vi "Periodic Tasks.vi"(8 "error in":errorcluster) -> ()   [LabVIEW 2015]
doc: "This VI runs in parallel to other tasks. It can contain as many user-defined periodic loops as you need. These can carry out PID or other sorts of timed response."
uses:
  <vilib>/Rock Robotics/WPI/Solenoid/WPI_SolenoidValue.ctl
  Robot Global Data.vi
  <vilib>/Rock Robotics/Network Tables/NT Write Raw.vi
  <vilib>/Rock Robotics/Network Tables/NT Write Boolean.vi
  <vilib>/Rock Robotics/WPI/Solenoid/WPI_SolenoidSetEnum.vi
  <vilib>/Rock Robotics/Network Tables/NT Write Number.vi
  <vilib>/Rock Robotics/Network Tables/NT Write Numeric Array.vi
  <vilib>/Rock Robotics/Network Tables/NT Read Boolean.vi
  <vilib>/Rock Robotics/WPI/Utilities/WPI_GetSetVariantRefNum.vi
panel:
  in  "Trim Speed":dbl
  in  "Rate":dbl min=0.0 max=0.1 step=0.001
  out "Ramp Up":dbl(knob) scale=0.0..1.0
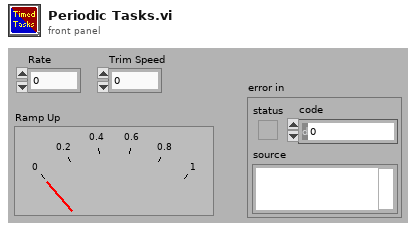
[diagram p1: front panel]
types:
  T1 = typedef "WPI_SolenoidValue.ctl" = enum16{"Off", "On", "Forward", "Reverse"}
  T2 = typedef "WPI_MotorControlDeviceRef.ctl" = cluster{"DeviceStatus":errorcluster, "Type":T3, "PWM":cluster{"PWM Channel":T4, "DeadBand":T5}, "CAN":cluster{"Device Number":u8, "Control Mode":T6, "Semaphore":T7, "Max Vout":dbl, "TalonSRX Control Mode":T8}, "Invert":bool}
  T3 = typedef "WPI_MotorControlType.ctl" = enum16{"PWM", "CAN", "CANTalonSRX"}
  T4 = typedef "FPGA_DIOPWMChannel.ctl" = enum8{"PWM 0", "PWM 1", "PWM 2", "PWM 3", "PWM 4", "PWM 5", "PWM 6", "PWM 7", "PWM 8", "PWM 9", "PWM MXP 0", "PWM MXP 1", "PWM MXP 2", "PWM MXP 3", "PWM MXP 4", "PWM MXP 5", "PWM MXP 6", "PWM MXP 7", "PWM MXP 8", "PWM MXP 9", "Invalid"}
  T5 = typedef "WPI_PWMDeadband.ctl" = cluster{"Name":string, "maxPositivePwm":i32, "minPositivePwm":i32, "centerPwm":i32, "maxNegativePwm":i32, "minNegativePwm":i32, "angularRange":u16}
  T6 = typedef "WPI_CANJaguar_ControlMode.ctl" = enum8{"Percent VBus", "Current", "Speed", "Position", "Voltage"}
  T7 = typedef "Semaphore RefNum" = refnum<k1>
  T8 = typedef "WPI_CANTalonSRX_APIControlMode.ctl" = enum8{"Percent VBus", "Speed", "Position", "Slave", "Unchanged / Invalid", "Voltage Compensation", "Current", "Motion Profile"}
  T9 = typedef "WPI_SolenoidDevRef.ctl" = cluster{"DevStatus":errorcluster, "Pneumatics Control Module":u8, "Forward Solenoid Channel":T10, "Reverse Solenoid Channel":T10}
  T10 = typedef "WPI_SolenoidChannel.ctl" = enum8{"Solenoid 0", "Solenoid 1", "Solenoid 2", "Solenoid 3", "Solenoid 4", "Solenoid 5", "Solenoid 6", "Solenoid 7", "Invalid"}
  T11 = typedef "WPI_DigitalInputDevRef.ctl" = cluster{"DevStatus":errorcluster, "DIO Channel":T12}
  T12 = typedef "FPGA_DIOChannel.ctl" = enum8{"DIO 0", "DIO 1", "DIO 2", "DIO 3", "DIO 4", "DIO 5", "DIO 6", "DIO 7", "DIO 8", "DIO 9", "DIO MXP 0", "DIO MXP 1", "DIO MXP 2", "DIO MXP 3", "DIO MXP 4", "DIO MXP 5", "DIO MXP 6", "DIO MXP 7", "DIO MXP 8", "DIO MXP 9", "DIO MXP 10", "DIO MXP 11", "DIO MXP 12", "DIO MXP 13", "DIO MXP 14", "DIO MXP 15", "Invalid"}
  T13 = typedef "WPI_RobotDriveDevRef.ctl" = cluster{"DevStatus":errorcluster, "Motors[]":T2[], "Square Inputs":bool, "Max Output":dbl}
  T14 = typedef "WPI_DriverStationRobotMode2.ctl" = enum16{"Autonomous Disabled", "Autonomous Enabled", "Teleop Disabled", "Teleop Enabled", "Disconnected", "Finish", "Test Disabled", "Test Enabled", "Emergency Stopped"}
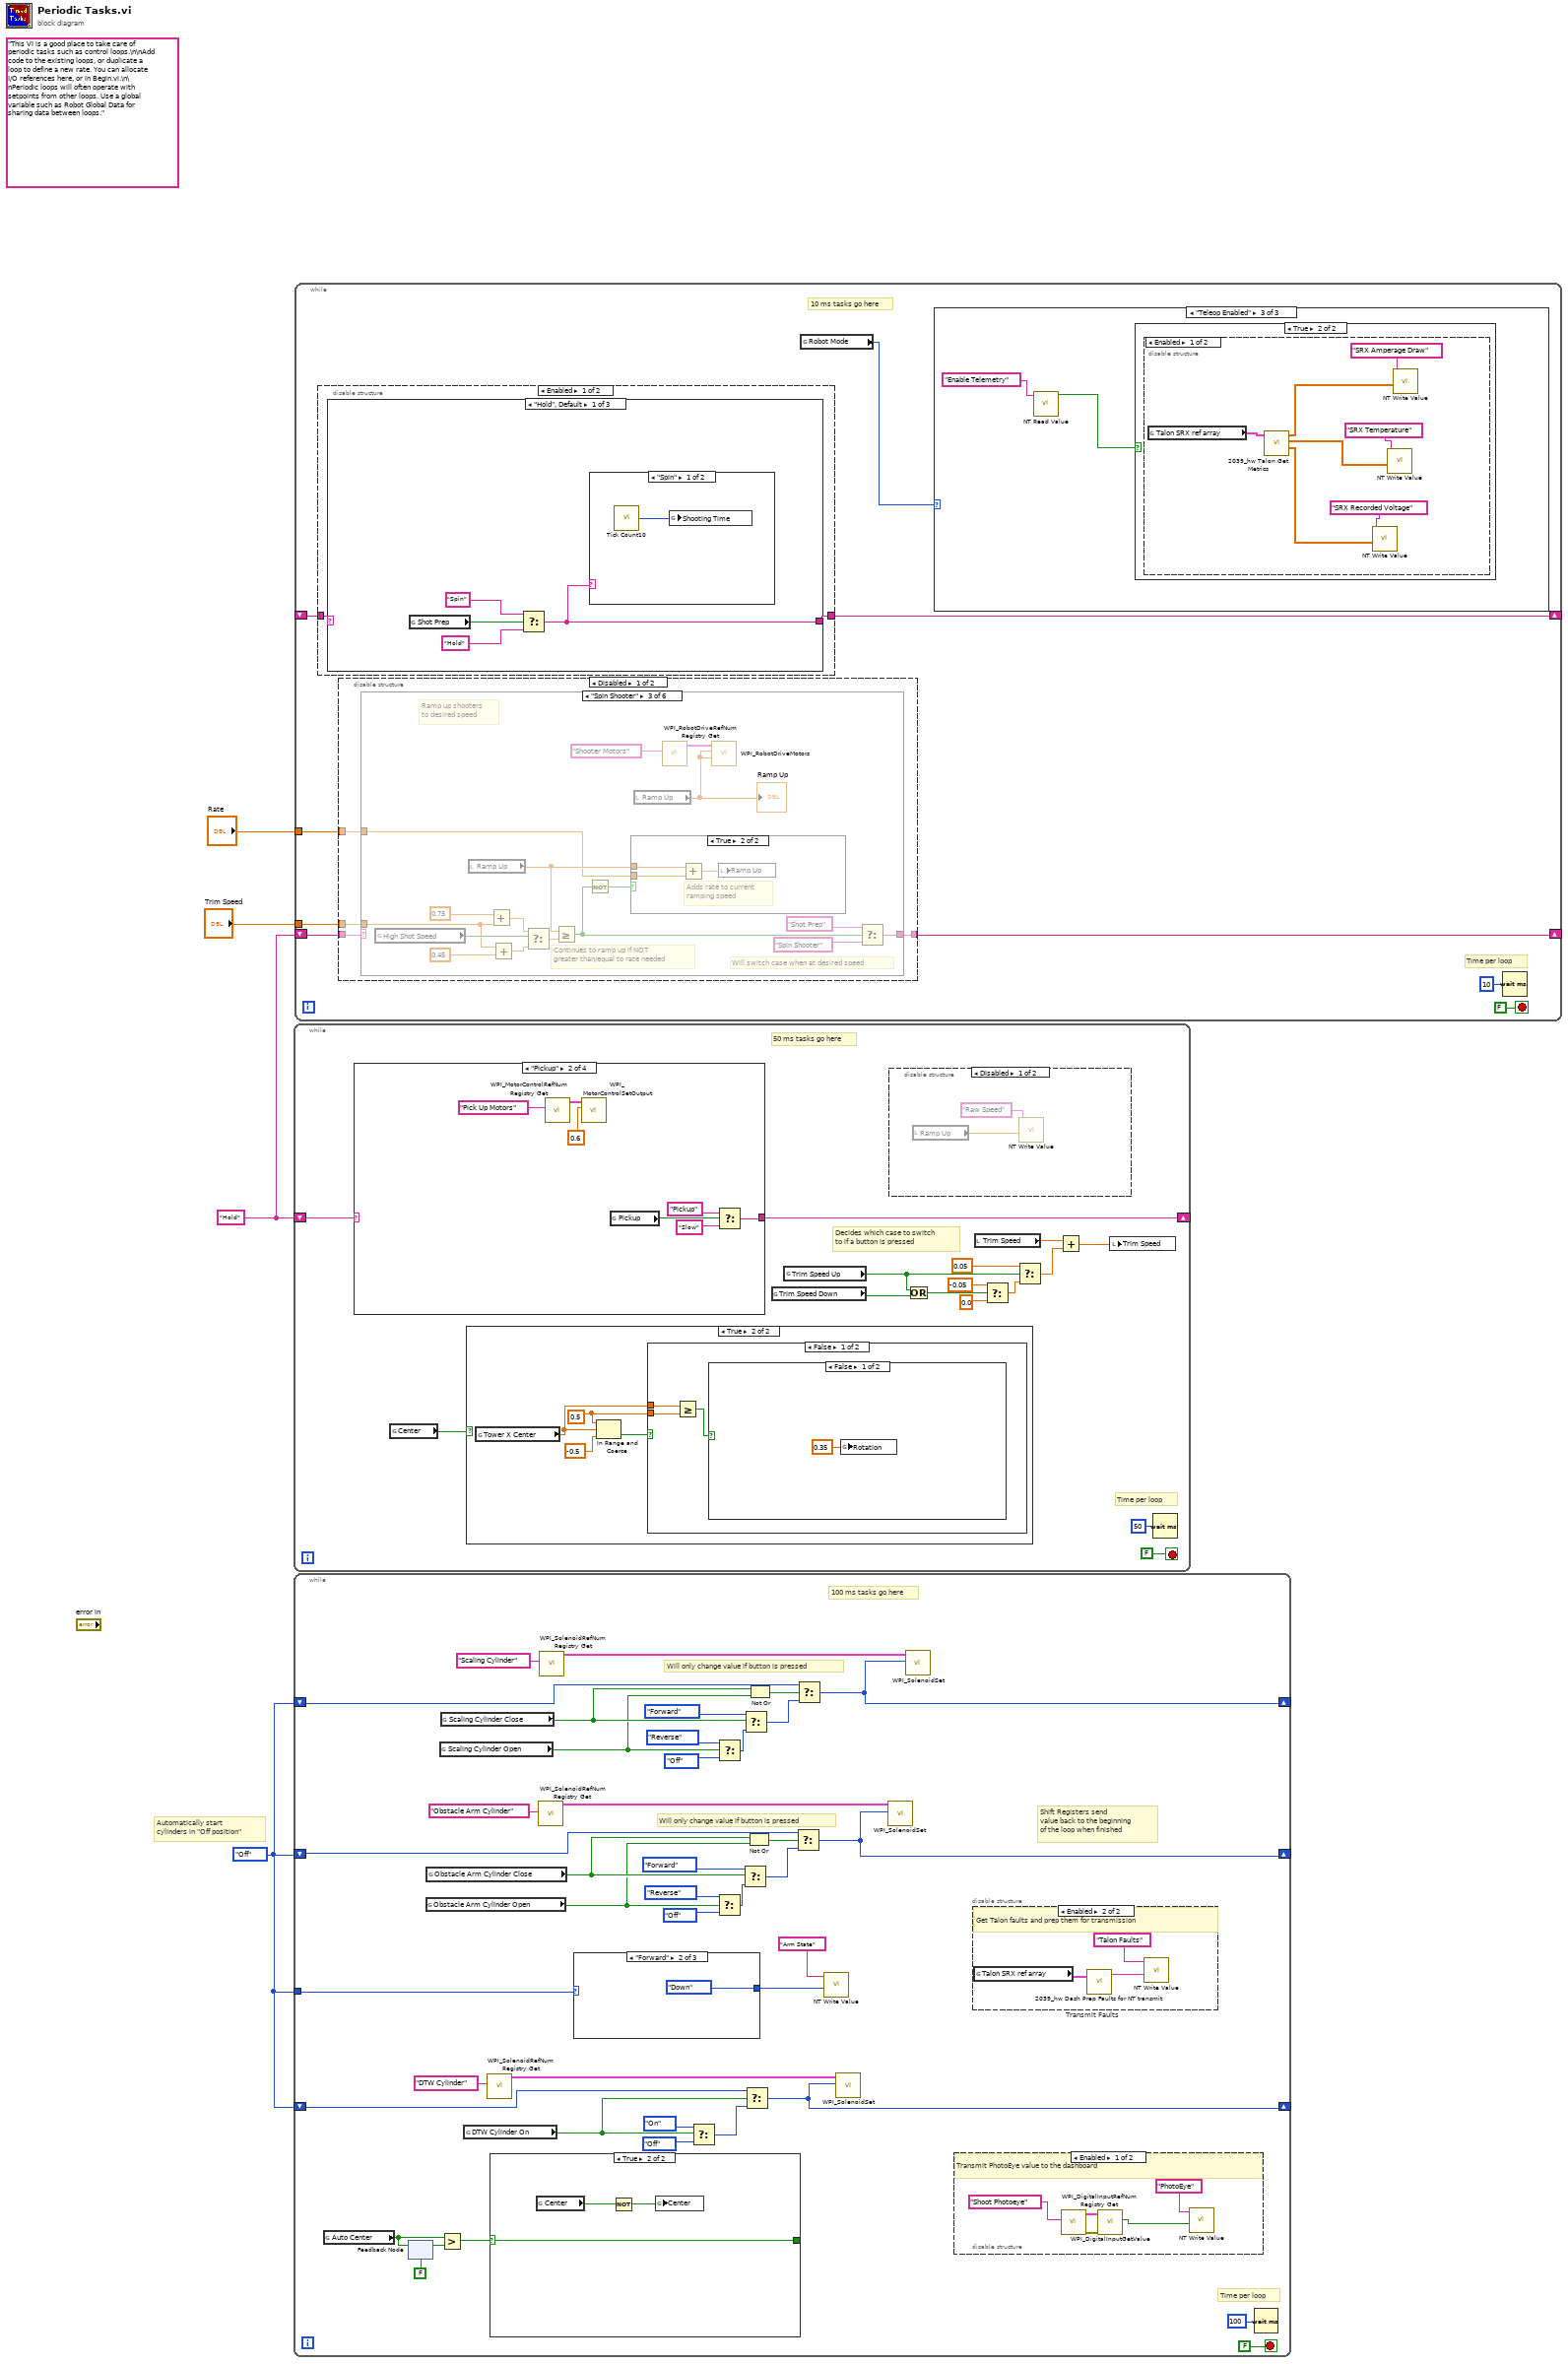
[diagram p0: block diagram]
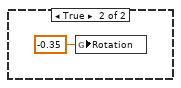
[diagram p4: hidden frame]
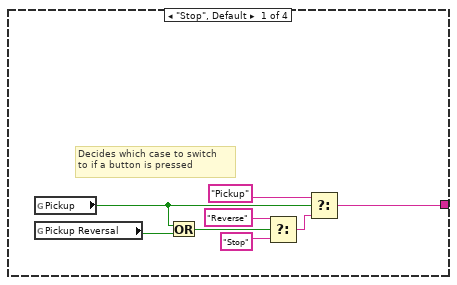
[diagram p6: hidden frame]
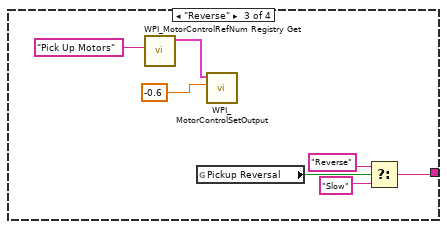
[diagram p7: hidden frame]
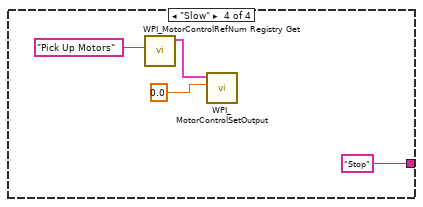
[diagram p8: hidden frame]
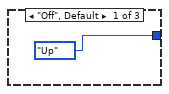
[diagram p11: hidden frame]
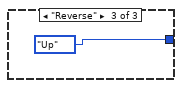
[diagram p12: hidden frame]
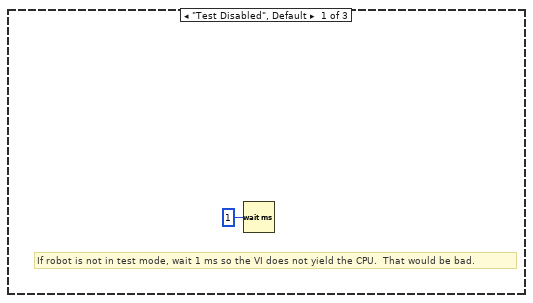
[diagram p14: hidden frame]
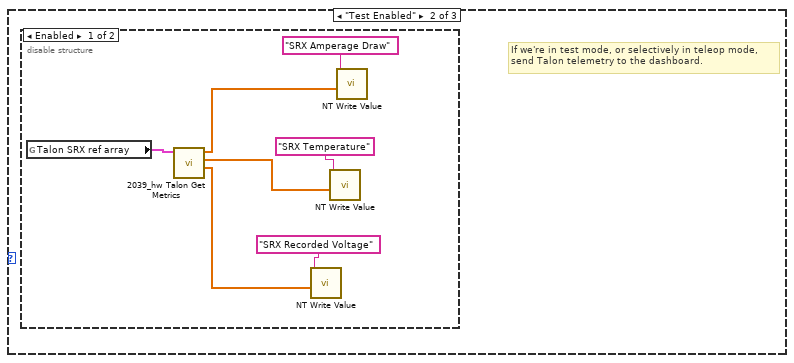
[diagram p15: hidden frame]
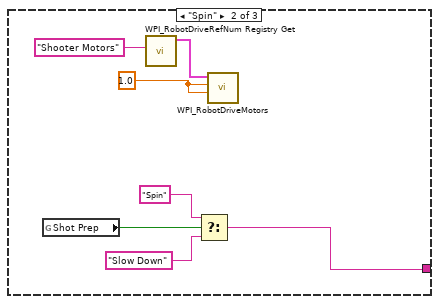
[diagram p20: hidden frame]
diagram:
  w1 = WPI_SolenoidValue."Off" ("Value")
  w3 = "Hold"
  (unwired) "This VI is a good place to take care of periodic tasks such as control loops.\n\nAdd code to the existing loops, or duplicate a loop to define a new rate. You can allocate I/O references here, or in Begin.vi.\n\nPeriodic loops will often operate with setpoints from other loops. Use a global variable such as Robot Global Data for sharing data between loops."
  # "Automatically start \ncylinders in \"Off position\""
  n1 = while {
    shift-right: [w16] -> _
    shift-left: w3 -> [w17]
    stop <- FALSE stop-if-true
    # "Decides which case to switch \nto if a button is pressed"
    # "Time per loop"
    # "50 ms tasks go here"
    n2 = case shown="\"Pickup\"" w17 {
      tunnel: [w31 w42 w47 "Stop" ("f")] -> w16
      frame "Stop", Default {
        # "Decides which case to switch \nto if a button is pressed"
        n3 = global read "Robot Global Data.vi" "Pickup"() -> (w33:bool)
        n4 = global read "Robot Global Data.vi" "Pickup Reversal"() -> (w32:bool)
        n5 = Or(x=w33, y=w32) -> (x .or. y?=w34:bool)
        n6 = Select(t="Reverse", s=w34, f="Stop") -> (s? t:f=w38:string)
        n7 = Select(t="Pickup", s=w33, f=w38) -> (s? t:f=w31:string)
      }
      frame "Pickup" {
        n8 = call <vilib>:"WPI_MotorControlRefNum Registry Get.vi"("refnum name"="Pick Up Motors") -> ("MotorControlDevRef"=w39:T2)  [unwired: 9 in, 1 out]
        n9 = call <vilib>:"WPI_MotorControlSetOutput.vi"("Output"=0.6 ("RightSpeed"), "MotorControlDevRef"=w39) -> ()  [unwired: 7 in, 3 out]
        n10 = global read "Robot Global Data.vi" "Pickup"() -> (w44:bool)
        n11 = Select(t="Pickup", s=w44, f="Slow") -> (s? t:f=w42:string)
      }
      frame "Reverse" {
        n12 = call <vilib>:"WPI_MotorControlRefNum Registry Get.vi"("refnum name"="Pick Up Motors") -> ("MotorControlDevRef"=w46:T2)  [unwired: 9 in, 1 out]
        n13 = global read "Robot Global Data.vi" "Pickup Reversal"() -> (w49:bool)
        n14 = call <vilib>:"WPI_MotorControlSetOutput.vi"("Output"=-0.6 ("RightSpeed"), "MotorControlDevRef"=w46) -> ()  [unwired: 7 in, 3 out]
        n15 = Select(t="Reverse", s=w49, f="Slow") -> (s? t:f=w47:string)
      }
      frame "Slow" {
        n16 = call <vilib>:"WPI_MotorControlRefNum Registry Get.vi"("refnum name"="Pick Up Motors") -> ("MotorControlDevRef"=w53:T2)  [unwired: 9 in, 1 out]
        n17 = call <vilib>:"WPI_MotorControlSetOutput.vi"("Output"=0.0 ("RightSpeed"), "MotorControlDevRef"=w53) -> ()  [unwired: 7 in, 3 out]
      }
    }
    n18 = global read "Robot Global Data.vi" "Center"() -> (w5:bool)
    n19 = case shown="True" w5 {
      frame False {
      }
      frame True {
        w22 = 0.5 ("y")
        n20 = global read "Robot Global Data.vi" "Tower X Center"() -> (w24:dbl)
        n21 = In Range and Coerce(upper limit=w22, x=w24, lower limit=-0.5 ("y")) -> (In Range?=w23:bool)  [unwired: 1 out]
        n22 = case shown="False" w23 {
          tunnel: w24 -> [w27 _]
          tunnel: w22 -> [w26 _]
          frame False {
            n23 = Greater Or Equal?(x=w27, y=w26) -> (x >= y?=w28:bool)
            n24 = case shown="False" w28 {
              frame False {
                n25 = global write "Robot Global Data.vi" "Rotation"(0.35 ("Rotation")) -> ()
              }
              frame True {
                n26 = global write "Robot Global Data.vi" "Rotation"(-0.35 ("Rotation")) -> ()
              }
            }
          }
          frame True {
          }
        }
      }
    }
    n27 = global read "Robot Global Data.vi" "Trim Speed Down"() -> (w14:bool)
    n28 = global read "Robot Global Data.vi" "Trim Speed Up"() -> (w12:bool)
    n29 = disable-structure shown="Disabled" {
      frame Disabled {
        n30 = local read "Ramp Up"() -> (w20:dbl)
        n31 = call-poly <vilib>:"NT Write Value.vi"("Numeric"=w20, "Name"="Raw Speed") -> ()  [unwired: 9 in, 1 out]
      }
      frame Enabled {
      }
    }
    n32 = Or(x=w12, y=w14) -> (x .or. y?=w13:bool)
    n33 = local read "Trim Speed"() -> (w7:dbl)
    n34 = Select(t=-0.05, s=w13, f=0.0) -> (s? t:f=w15:dbl)
    n35 = Select(t=0.05, s=w12, f=w15) -> (s? t:f=w8:dbl)
    n36 = Add(x=w7, y=w8) -> (x+y=w6:dbl)
    n37 = local write "Trim Speed"(w6) -> ()
    n38 = Wait (ms)(milliseconds to wait=u32 50) -> ()  [unwired: 1 out]
  }
  n39 = while {
    shift-right: [w95] -> _
    shift-left: w1 -> [w94]
    shift-right: [w89] -> _
    shift-left: w1 -> [w90]
    shift-right: [w85] -> _
    shift-left: w1 -> [w84]
    tunnel: w1 -> [w63]
    stop <- FALSE stop-if-true
    # "Will only change value if button is pressed"
    # "Will only change value if button is pressed"
    # "Shift Registers send\nvalue back to the beginning\nof the loop when finished"
    # "Time per loop"
    # "100 ms tasks go here"
    n40 = global read "Robot Global Data.vi" "Auto Center"() -> (w58:bool)
    n41 = feedback-in #1(w58) -> ()
    n42 = feedback #1(FALSE ("Auto Center")) -> (w59:bool)
    n43 = global read "Robot Global Data.vi" "Obstacle Arm Cylinder Open"() -> (w74:bool)
    n44 = global read "Robot Global Data.vi" "Obstacle Arm Cylinder Close"() -> (w75:bool)
    n45 = global read "Robot Global Data.vi" "Scaling Cylinder Open"() -> (w64:bool)
    n46 = Greater?(x=w58, y=w59) -> (0:w60:bool)
    n47 = global read "Robot Global Data.vi" "Scaling Cylinder Close"() -> (w65:bool)
    n48 = global read "Robot Global Data.vi" "DTW Cylinder On"() -> (w86:bool)
    n49 = call <vilib>:"WPI_SolenoidRefNum Registry Get.vi"("refnum name"="DTW Cylinder") -> ("SolenoidDevRef"=w92:T9)  [unwired: 9 in, 1 out]
    n50 = case shown="True" w60 {
      selector: w60 -> [w109 w112]
      tunnel: [w109 w112] -> _
      frame False {
      }
      frame True {
        n51 = global read "Robot Global Data.vi" "Center"() -> (w110:bool)
        n52 = Not(x=w110) -> (.not. x?=w111:bool)
        n53 = global write "Robot Global Data.vi" "Center"(w111) -> ()
      }
    }
    n54 = call <vilib>:"WPI_SolenoidRefNum Registry Get.vi"("refnum name"="Obstacle Arm Cylinder") -> ("SolenoidDevRef"=w78:T9)  [unwired: 9 in, 1 out]
    n55 = call <vilib>:"WPI_SolenoidRefNum Registry Get.vi"("refnum name"="Scaling Cylinder") -> ("SolenoidDevRef"=w68:T9)  [unwired: 9 in, 1 out]
    n56 = case shown="\"Forward\"" w63 {
      tunnel: [enum16{"Up", "Down"}."Up" enum16{"Up", "Down"}."Down" enum16{"Up", "Down"}."Up"] -> w62
      frame "Off", Default {
      }
      frame "Forward" {
      }
      frame "Reverse" {
      }
    }
    n57 = Select(t=WPI_SolenoidValue."On" ("Value"), s=w86, f=WPI_SolenoidValue."Off" ("Value")) -> (s? t:f=w91:T1)
    n58 = Select(t=WPI_SolenoidValue."Reverse" ("Value"), s=w74, f=WPI_SolenoidValue."Off" ("Value")) -> (s? t:f=w80:T1)
    n59 = Select(t=WPI_SolenoidValue."Reverse" ("Value"), s=w64, f=WPI_SolenoidValue."Off" ("Value")) -> (s? t:f=w70:T1)
    n60 = Select(t=WPI_SolenoidValue."Forward" ("Value"), s=w75, f=w80) -> (s? t:f=w77:T1)
    n61 = Select(t=WPI_SolenoidValue."Forward" ("Value"), s=w65, f=w70) -> (s? t:f=w67:T1)
    n62 = Select(t=w90, s=w86, f=w91) -> (s? t:f=w89:T1)
    n63 = Not Or(1:w74, 2:w75) -> (0:w76:bool)
    n64 = Not Or(1:w64, 2:w65) -> (0:w66:bool)
    n65 = Select(t=w84, s=w76, f=w77) -> (s? t:f=w85:T1)
    n66 = Select(t=w94, s=w66, f=w67) -> (s? t:f=w95:T1)
    n67 = call-poly <vilib>:"NT Write Value.vi"("Numeric"=w62, "Name"="Arm State") -> ()  [unwired: 9 in, 1 out]
    n68 = call-poly <vilib>:"WPI_SolenoidSet.vi"("Value"=w89, "SolenoidDevRef"=w92) -> ()  [unwired: 1 in, 9 out]
    n69 = call-poly <vilib>:"WPI_SolenoidSet.vi"("Value"=w85, "SolenoidDevRef"=w78) -> ()  [unwired: 1 in, 9 out]
    n70 = call-poly <vilib>:"WPI_SolenoidSet.vi"("Value"=w95, "SolenoidDevRef"=w68) -> ()  [unwired: 1 in, 9 out]
    n71 = disable-structure shown="Enabled" {
      frame Enabled {
        # "Transmit PhotoEye value to the dashboard"
        n72 = call <vilib>:"WPI_DigitalInputRefNum Registry Get.vi"("refnum name"="Shoot Photoeye") -> ("error out"=w100:errorcluster, "DigitalInputDevRef"=w101:T11)  [unwired: 9 in]
        n73 = call <vilib>:"WPI_DigitalInputGetValue.vi"("error in (no error)"=w100, "DigitalInputDevRef"=w101) -> ("Value"=w99:bool)  [unwired: 7 in, 2 out]
        n74 = call-poly <vilib>:"NT Write Value.vi"("Boolean"=w99, "Name"="PhotoEye") -> ()  [unwired: 9 in, 1 out]
      }
      frame Disabled {
      }
    }
    n75 = disable-structure "Transmit Faults" shown="Enabled" {
      frame Disabled {
      }
      frame Enabled {
        # "Get Talon faults and prep them for transmission"
        n76 = global read "Robot Global Data.vi" "Talon SRX ref array"() -> (w105:T2[])
        n77 = call "2039_hw Dash Prep Faults for NT transmit.vi"("Talon SRX ref array"=w105) -> ("data string"=w103:string)  [unwired: 1 in, 1 out]
        n78 = call-poly <vilib>:"NT Write Value.vi"("Raw"=w103, "Name"="Talon Faults") -> ()  [unwired: 9 in, 1 out]
      }
    }
    n79 = Wait (ms)(milliseconds to wait=u32 100) -> ()  [unwired: 1 out]
  }
  n80 = while {
    shift-right: [w119] -> _
    shift-left: _ -> [w115]
    tunnel: "Rate" -> [w118]
    shift-right: [w117] -> _
    shift-left: w3 -> [w116]
    tunnel: "Trim Speed" -> [w114]
    stop <- FALSE stop-if-true
    # "10 ms tasks go here"
    # "Time per loop"
    n81 = disable-structure shown="Enabled" {
      disable-tunnel: [w140 _] -> w119
      disable-tunnel: w115 -> [w139 _]
      frame Enabled {
        n82 = case shown="\"Hold\", Default" w139 {
          tunnel: [w141 w150 w153] -> w140
          frame "Hold", Default {
            n83 = global read "Robot Global Data.vi" "Shot Prep"() -> (w144:bool)
            n84 = Select(t="Spin", s=w144, f="Hold") -> (s? t:f=w141:string)
            n85 = case shown="\"Spin\"" w141 {
              frame "Spin" {
                n86 = call "Tick Count10"() -> ("Tick Count(mSec)"=w145:u32)
                n87 = global write "Robot Global Data.vi" "Shooting Time"(w145) -> ()
              }
              frame "Hold", Default {
              }
            }
          }
          frame "Spin" {
            w146 = 1.0 ("RightSpeed")
            n88 = global read "Robot Global Data.vi" "Shot Prep"() -> (w149:bool)
            n89 = call <vilib>:"WPI_RobotDriveRefNum Registry Get.vi"("refnum name"="Shooter Motors") -> ("RobotDriveDevRef"=w147:T13)  [unwired: 9 in, 1 out]
            n90 = Select(t="Spin", s=w149, f="Slow Down") -> (s? t:f=w150:string)
            n91 = call <vilib>:"WPI_RobotDriveMotors.vi"("RightSpeed"=w146, "LeftSpeed"=w146, "RobotDriveDevRef"=w147) -> ()  [unwired: 6 in, 3 out]
          }
          frame "Slow Down" {
            w161 = 0.0 ("RightSpeed")
            n92 = global read "Robot Global Data.vi" "Shooting Time"() -> (w154:i32)
            n93 = call "Tick Count14"() -> ("Tick Count(mSec)"=w155:u32)
            n94 = Subtract(x=w155, y=w154) -> (x-y=w158:u32)
            n95 = call <vilib>:"WPI_RobotDriveRefNum Registry Get.vi"("refnum name"="Shooter Motors") -> ("RobotDriveDevRef"=w162:T13)  [unwired: 9 in, 1 out]
            n96 = call <vilib>:"WPI_RobotDriveMotors.vi"("RightSpeed"=w161, "LeftSpeed"=w161, "RobotDriveDevRef"=w162) -> ()  [unwired: 6 in, 3 out]
            n97 = Greater?(x=w158, y=u32 10) -> (0:w159:bool)
            n98 = Select(t="Hold", s=w159, f="Slow Down") -> (s? t:f=w153:string)
          }
        }
      }
      frame Disabled {
      }
    }
    n99 = disable-structure shown="Disabled" {
      disable-tunnel: w118 -> [w167 _]
      disable-tunnel: [w166 _] -> w117
      disable-tunnel: w116 -> [w165 _]
      disable-tunnel: w114 -> [w164 _]
      frame Disabled {
        n100 = case shown="\"Spin Shooter\"" w165 {
          tunnel: [w168 w176 w196 w206 w213 "Hold" ("t")] -> w166
          tunnel: w167 -> [_ _ w192 _ _ _]
          tunnel: w164 -> [_ _ w186 _ _ _]
          frame "Hold", Default {
            # "Ball being held inside robot \n(probably between shooters)"
            n101 = global read "Robot Global Data.vi" "Shot Prep"() -> (w171:bool)
            n102 = Select(t="Spin Shooter", s=w171, f="Hold") -> (s? t:f=w168:string)
            n103 = case shown="\"Spin Shooter\"" w168 {
              frame "Spin Shooter" {
                # "When shot process is \nstarted, timer starts"
                n104 = call "Tick Count"() -> ("Tick Count(mSec)"=w172:u32)
                n105 = global write "Robot Global Data.vi" "Shooting Time"(w172) -> ()
              }
              frame "Hold", Default {
                # "Do Nothing"
              }
            }
          }
          frame "Unload Ball" {
            w173 = -0.1 ("RightSpeed")
            # "Move ball out of \nshooters before spinup"
            n106 = global read "Robot Global Data.vi" "Shooting Time"() -> (w177:i32)
            n107 = call <vilib>:"WPI_RobotDriveRefNum Registry Get.vi"("refnum name"="Shooter Motors") -> ("RobotDriveDevRef"=w174:T13)  [unwired: 9 in, 1 out]
            n108 = call "Tick Count2"() -> ("Tick Count(mSec)"=w178:u32)
            n109 = Subtract(x=w178, y=w177) -> (x-y=w181:u32)
            n110 = call <vilib>:"WPI_RobotDriveMotors.vi"("RightSpeed"=w173, "LeftSpeed"=w173, "RobotDriveDevRef"=w174) -> ()  [unwired: 6 in, 3 out]
            n111 = Greater?(x=w181, y=u32 250) -> (0:w182:bool)
            n112 = Select(t="Spin Shooter", s=w182, f="Unload Ball") -> (s? t:f=w176:string)
          }
          frame "Spin Shooter" {
            # "Ramp up shooters\nto desired speed"
            # "Will switch case when at desired speed"
            # "Continues to ramp up if NOT \ngreater than/equal to rate needed"
            n113 = global read "Robot Global Data.vi" "High Shot Speed"() -> (w190:bool)
            n114 = local read "Ramp Up"() -> (w195:dbl)
            n115 = Add(x=0.75 ("y"), y=w186) -> (x+y=w188:dbl)
            n116 = Add(x=w186, y=0.45) -> (x+y=w187:dbl)
            n117 = Select(t=w188, s=w190, f=w187) -> (s? t:f=w191:dbl)
            n118 = Greater Or Equal?(x=w195, y=w191) -> (x >= y?=w193:bool)
            n119 = Not(x=w193) -> (.not. x?=w194:bool)
            n120 = case shown="True" w194 {
              tunnel: w192 -> [_ w204]
              tunnel: w195 -> [_ w203]
              frame False {
                # "If at correct speed, stay at that speed"
                n121 = local read "Ramp Up"() -> (w201:dbl)
                n122 = local write "Ramp Up"(w201) -> ()
              }
              frame True {
                # "Adds rate to current \nramping speed"
                n123 = Add(x=w203, y=w204) -> (x+y=w202:dbl)
                n124 = local write "Ramp Up"(w202) -> ()
              }
            }
            n125 = local read "Ramp Up"() -> (w189:dbl)
            "Ramp Up" <- w189
            n126 = call <vilib>:"WPI_RobotDriveRefNum Registry Get.vi"("refnum name"="Shooter Motors") -> ("RobotDriveDevRef"=w197:T13)  [unwired: 9 in, 1 out]
            n127 = call <vilib>:"WPI_RobotDriveMotors.vi"("RightSpeed"=w189, "LeftSpeed"=w189, "RobotDriveDevRef"=w197) -> ()  [unwired: 6 in, 3 out]
            n128 = Select(t="Shot Prep", s=w193, f="Spin Shooter") -> (s? t:f=w196:string)
          }
          frame "Shot Prep" {
            # "Added to allow you to stop the \nspinup process midway if needed"
            n129 = global read "Robot Global Data.vi" "Shot Prep"() -> (w207:bool)
            n130 = global read "Robot Global Data.vi" "Pickup"() -> (w205:bool)
            n131 = Or(x=w205, y=w207) -> (x .or. y?=w208:bool)
            n132 = Select(t="Slow Down", s=w208, f="Shot Prep") -> (s? t:f=w212:string)
            n133 = Select(t="Take Shot", s=w205, f=w212) -> (s? t:f=w206:string)
          }
          frame "Take Shot" {
            w222 = 0.6 ("RightSpeed")
            # "Slow down after 750ms"
            # "Throws the ball through\nshooter motors"
            n134 = global read "Robot Global Data.vi" "Shooting Time"() -> (w215:i32)
            n135 = call "Tick Count3"() -> ("Tick Count(mSec)"=w216:u32)
            n136 = call <vilib>:"WPI_RobotDriveRefNum Registry Get.vi"("refnum name"="Shooter Motors") -> ("RobotDriveDevRef"=w221:T13)  [unwired: 9 in, 1 out]
            n137 = Subtract(x=w216, y=w215) -> (x-y=w218:u32)
            n138 = call <vilib>:"WPI_RobotDriveMotors.vi"("RightSpeed"=w222, "LeftSpeed"=w222, "RobotDriveDevRef"=w221) -> ()  [unwired: 6 in, 3 out]
            n139 = Greater?(x=w218, y=u32 750) -> (0:w219:bool)
            n140 = Select(t="Slow Down", s=w219, f="Take Shot") -> (s? t:f=w213:string)
          }
          frame "Slow Down" {
            w227 = 0.0 ("RightSpeed")
            # "Slow down the\nmotors to 0"
            n141 = call <vilib>:"WPI_RobotDriveRefNum Registry Get.vi"("refnum name"="Shooter Motors") -> ("RobotDriveDevRef"=w226:T13)  [unwired: 9 in, 1 out]
            n142 = call <vilib>:"WPI_RobotDriveMotors.vi"("RightSpeed"=w227, "LeftSpeed"=w227, "RobotDriveDevRef"=w226) -> ()  [unwired: 6 in, 3 out]
          }
        }
      }
      frame Enabled {
      }
    }
    n143 = global read "Robot Global Data.vi" "Robot Mode"() -> (w113:T14)
    n144 = case shown="\"Teleop Enabled\"" w113 {
      frame "Test Disabled", Default {
        # "If robot is not in test mode, wait 1 ms so the VI does not yield the CPU.  That would be bad."
        n145 = Wait (ms)(milliseconds to wait=u32 1) -> ()  [unwired: 1 out]
      }
      frame "Test Enabled" {
        # "If we're in test mode, or selectively in teleop mode,\nsend Talon telemetry to the dashboard."
        n146 = disable-structure shown="Enabled" {
          frame Enabled {
            n147 = global read "Robot Global Data.vi" "Talon SRX ref array"() -> (w123:T2[])
            n148 = call "2039_hw Talon Get Metrics.vi"("Talon SRX ref array"=w123) -> ("Vbat"=w129:dbl[], "Temperature"=w127:dbl[], "Amperage Draw"=w125:dbl[])  [unwired: 8 in]
            n149 = call-poly <vilib>:"NT Write Value.vi"("Numeric Array"=w129, "Name"="SRX Recorded Voltage") -> ()  [unwired: 9 in, 1 out]
            n150 = call-poly <vilib>:"NT Write Value.vi"("Numeric Array"=w127, "Name"="SRX Temperature") -> ()  [unwired: 9 in, 1 out]
            n151 = call-poly <vilib>:"NT Write Value.vi"("Numeric Array"=w125, "Name"="SRX Amperage Draw") -> ()  [unwired: 9 in, 1 out]
          }
          frame Disabled {
          }
        }
      }
      frame "Teleop Enabled" {
        n152 = call-poly <vilib>:"NT Read Value.vi"("Name"="Enable Telemetry") -> ("Boolean"=w130:bool)  [unwired: 9 in, 1 out]
        n153 = case shown="True" w130 {
          frame False {
          }
          frame True {
            n154 = disable-structure shown="Enabled" {
              frame Enabled {
                n155 = global read "Robot Global Data.vi" "Talon SRX ref array"() -> (w132:T2[])
                n156 = call "2039_hw Talon Get Metrics.vi"("Talon SRX ref array"=w132) -> ("Vbat"=w138:dbl[], "Temperature"=w136:dbl[], "Amperage Draw"=w134:dbl[])  [unwired: 8 in]
                n157 = call-poly <vilib>:"NT Write Value.vi"("Numeric Array"=w138, "Name"="SRX Recorded Voltage") -> ()  [unwired: 9 in, 1 out]
                n158 = call-poly <vilib>:"NT Write Value.vi"("Numeric Array"=w136, "Name"="SRX Temperature") -> ()  [unwired: 9 in, 1 out]
                n159 = call-poly <vilib>:"NT Write Value.vi"("Numeric Array"=w134, "Name"="SRX Amperage Draw") -> ()  [unwired: 9 in, 1 out]
              }
              frame Disabled {
              }
            }
          }
        }
      }
    }
    n160 = Wait (ms)(milliseconds to wait=u32 10) -> ()  [unwired: 1 out]
  }
